vi "crdDisplayFit.vi"(6 "dt":dbl, 8 "N":i32=360, 9 "B":dbl, 10 "A":dbl, 11 "tau":dbl) -> (3 "Fit Out":dbl[](array[numeric]))   [LabVIEW 2011]
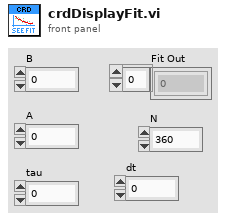
[diagram p1: front panel]
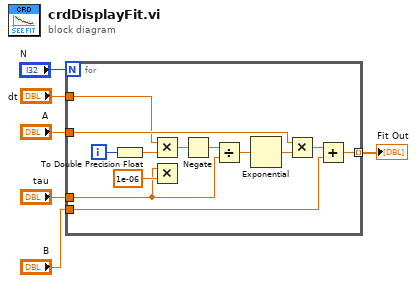
[diagram p0: block diagram]
diagram:
  n1 = for {
    N: "N" -> [_]
    tunnel: "A" -> [w19]
    tunnel: "B" -> [w13]
    tunnel: "tau" -> [w8]
    tunnel: [w12] -> w6 mode=indexing
    tunnel: "dt" -> [w7]
    i -> [w10]
    n2 = To Double Precision Float(number=w10) -> (double precision float=w9:dbl)
    n3 = Multiply(x=w7, y=w9) -> (x*y=w18:dbl)
    n4 = Multiply(x=w8, y=1e-06 ("x")) -> ()  [unwired: 1 out]
    n5 = Negate(x=w18) -> (-x=w17:dbl)
    n6 = Divide(x=w17, y=w8) -> (x/y=w16:dbl)
    n7 = Exponential(1:w16) -> (0:w15:dbl)
    n8 = Multiply(x=w19, y=w15) -> (x*y=w14:dbl)
    n9 = Add(x=w14, y=w13) -> (x+y=w12:dbl)
  }
  "Fit Out" <- w6
